vi "Read datatype.vi"(8 "error in (no error)":errorcluster, 11 "JSON Value in":refnum<class "JSON Value.lvclass">) -> (0 "error out":errorcluster, 2 "datatype":T1, 3 "JSON Value out":refnum<class "JSON Value.lvclass">)   [LabVIEW 2016, in "JSON Value.lvclass"]
doc: "Returns the JSON Type of the given object. This may be used to determine if the value of a control of type JSON Null, JSON Literal or JSON Structured Type is an instance of a more specific type."
uses:
  JSON Value.lvclass
  JSON Types.ctl
  JSON Value.lvclass/JSON Value.ctl
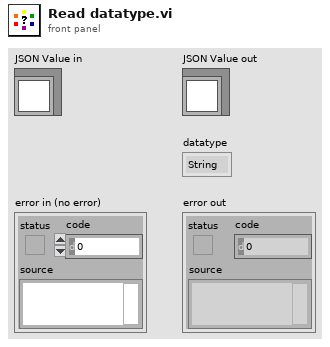
[diagram p1: front panel]
types:
  T1 = typedef "JSON Value.lvclass/JSON Types.ctl" = enum16{"String", "Numeric", "Boolean", "NULL", "Object", "Array"}
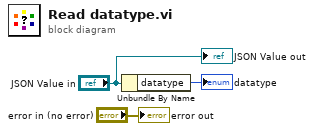
[diagram p0: block diagram]
diagram:
  n1 = Unbundle By Name("JSON Value in") -> ("datatype"=→"datatype":T1)
  "error out" <- "error in (no error)"
  "JSON Value out" <- "JSON Value in"
